vi "Close.vi"(8 "error in (no error)":errorcluster, 11 "Ref in":refnum<queue>) -> (0 "error out":errorcluster)   [LabVIEW 2016, in "SEQ.lvlib"]
doc: "Close the Single Element Queued based variable."
uses:
  SEQ.lvlib
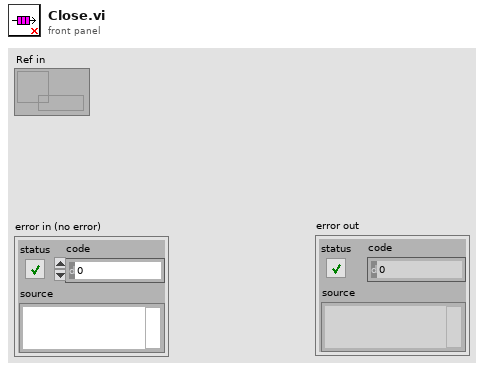
[diagram p1: front panel]
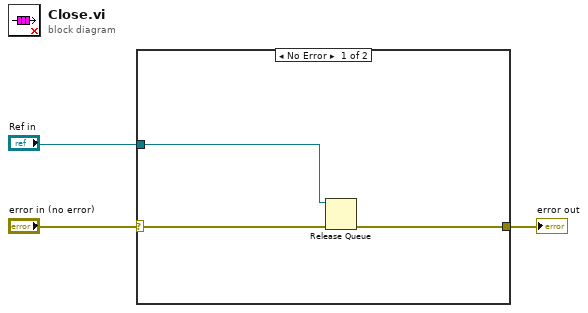
[diagram p0: block diagram]
diagram:
  n1 = case shown="No Error" "error in (no error)" {
    selector: "error in (no error)" -> [w6 w7]
    tunnel: [w5 w7] -> w2
    tunnel: "Ref in" -> [w4 _]
    frame No Error {
      n2 = Release Queue(queue=w4, error in (no error)=w6) -> (error out=w5:errorcluster)  [unwired: 1 in, 2 out]
    }
    frame Error {
    }
  }
  "error out" <- w2
